vi "Vector space kNN.vi"() -> ()   [LabVIEW 2014]
uses:
  <vilib>/Utility/file.llb/Write To Spreadsheet File (string).vi
panel:
  out "Array 4":string[][](array[string])
  out "Slide 2":dbl(slide) scale=0.0..204.0
  out "Slide":dbl(slide) scale=0.0..9.0
  in  "Path":path
  in  "all rows":string[][](array[string])=array2038x3[6114 elements]
  out "LCS/min (Lsample,Lknown)":dbl[][](array[numeric])
  out "Distance values (LCS)":dbl[][](array[numeric])
  out "size(s)":i32
  out "accuracy":string[][](array[string])
  out "Results":string[][](array[string])
  out "Training data (K)":string[][](array[string])
  out "test data K-1":string[][](array[string])
  in  "K folds K":i32=10
  out "K folds data":string[][](array[string])
  out "Assigned using LCS (enhanced)":string[][](array[string])
  out "Assigned using LCS":string[][](array[string])
  in  "class labels for training data":string[](array[string])
  in  "kNN k":i32=5
  in  "training data (cluster centers)":string[](array[string])
  in  "test data (patterns in)":string[](array[string])=["0 4 0", "4 0 4", "0 4 0", "4 0 4", "0 4 0", "4 0 4", "0 4 0", "4 0 -2", "0 -2 3", "-2 3 0", "3 0 3", "0 3 0", "3 0 4", "0 4 0", "-2 0 1", "0 1 0", "1 0 -4", "0 -4 4", "-2 2 0", "2 0 -1", "0 -1 -4", "-1 -4 1", "-4 1 0", "1 0 3", "0 3 0", "-1 0 -1", "0 -1 2", "0 -1 1", "-1 1 0", "1 0 4", "0 4 0", "4 0 3", "0 3 -2", "3 -2 0", "-2 0 -2", "0 -2 3", "-2 3 -2", "3 -2 0", "-2 0 4", "0 4 0", "4 0 -2", "0 -2 2", "2 -1 0", "-1 0 4", "0 4 0", "4 0 2", "0 2 0", "2 0 -2", "0 -2 0", "1 -1 0", "-1 0 3", "0 3 0", "3 0 -4", "0 -4 4", "-4 4 -4", "4 -4 0", "2 -1 0", "-1 0 3", "0 3 -2", "3 -2 0", "-2 0 -3", "0 -3 0", "-3 0 3", "0 3 0", "3 0 -3", "0 -3 0", "0 4 0", "4 0 4", "0 4 -4", "4 -4 1", "-4 1 -1", "1 -1 0", "-1 0 -3", "0 -3 0", "-3 0 1", "0 1 -4", "1 -4 1", "-4 1 0", "1 0 4", "0 4 0", "4 0 -4", "0 -4 0", "-4 0 -4", "0 -4 4", "-4 4 -4", "4 -4 1", "0 -4 1", "-4 1 0", "1 0 -4", "0 -4 4", "0 4 0", "4 0 -2", "0 -2 2", "-2 2 -2", "2 -2 2", "-2 2 -2", "2 -2 2", "-2 2 -1", "2 -1 0", "-1 0 4", "0 4 0", "4 0 2", "0 2 0", "2 0 4", "0 4 0", "4 0 2", "0 2 -2", "2 -2 0", "-2 0 4", "1 0 -1", "0 -1 0", "-1 0 -1", "0 -1 0", "-1 0 1", "0 1 -1", "-2 2 -2", "2 -2 3", "1 0 -1", "0 -1 0", "-1 0 -1", "0 -1 2", "-1 2 0", "2 0 2", "0 2 -2", "2 -2 0", "-2 0 -4", "0 -4 0", "-2 2 0", "2 0 3", "0 3 -2", "3 -2 2", "1 -1 0", "-1 0 3", "0 4 0", "-2 0 1", "0 1 -4", "1 -4 0", "-4 0 -3", "0 -3 0", "1 0 -1", "0 -1 2", "-1 2 -1", "2 -1 1", "-1 1 -4", "-2 0 -1", "0 -1 1", "0 3 0", "3 0 3", "0 3 0", "3 0 3", "0 3 -2", "-4 0 -4", "0 -4 4", "0 4 0", "4 0 -4", "0 -4 0", "-4 0 -4", "-2 2 0", "2 0 4", "0 4 -4", "4 -4 0", "-4 0 2", "0 2 -2"]
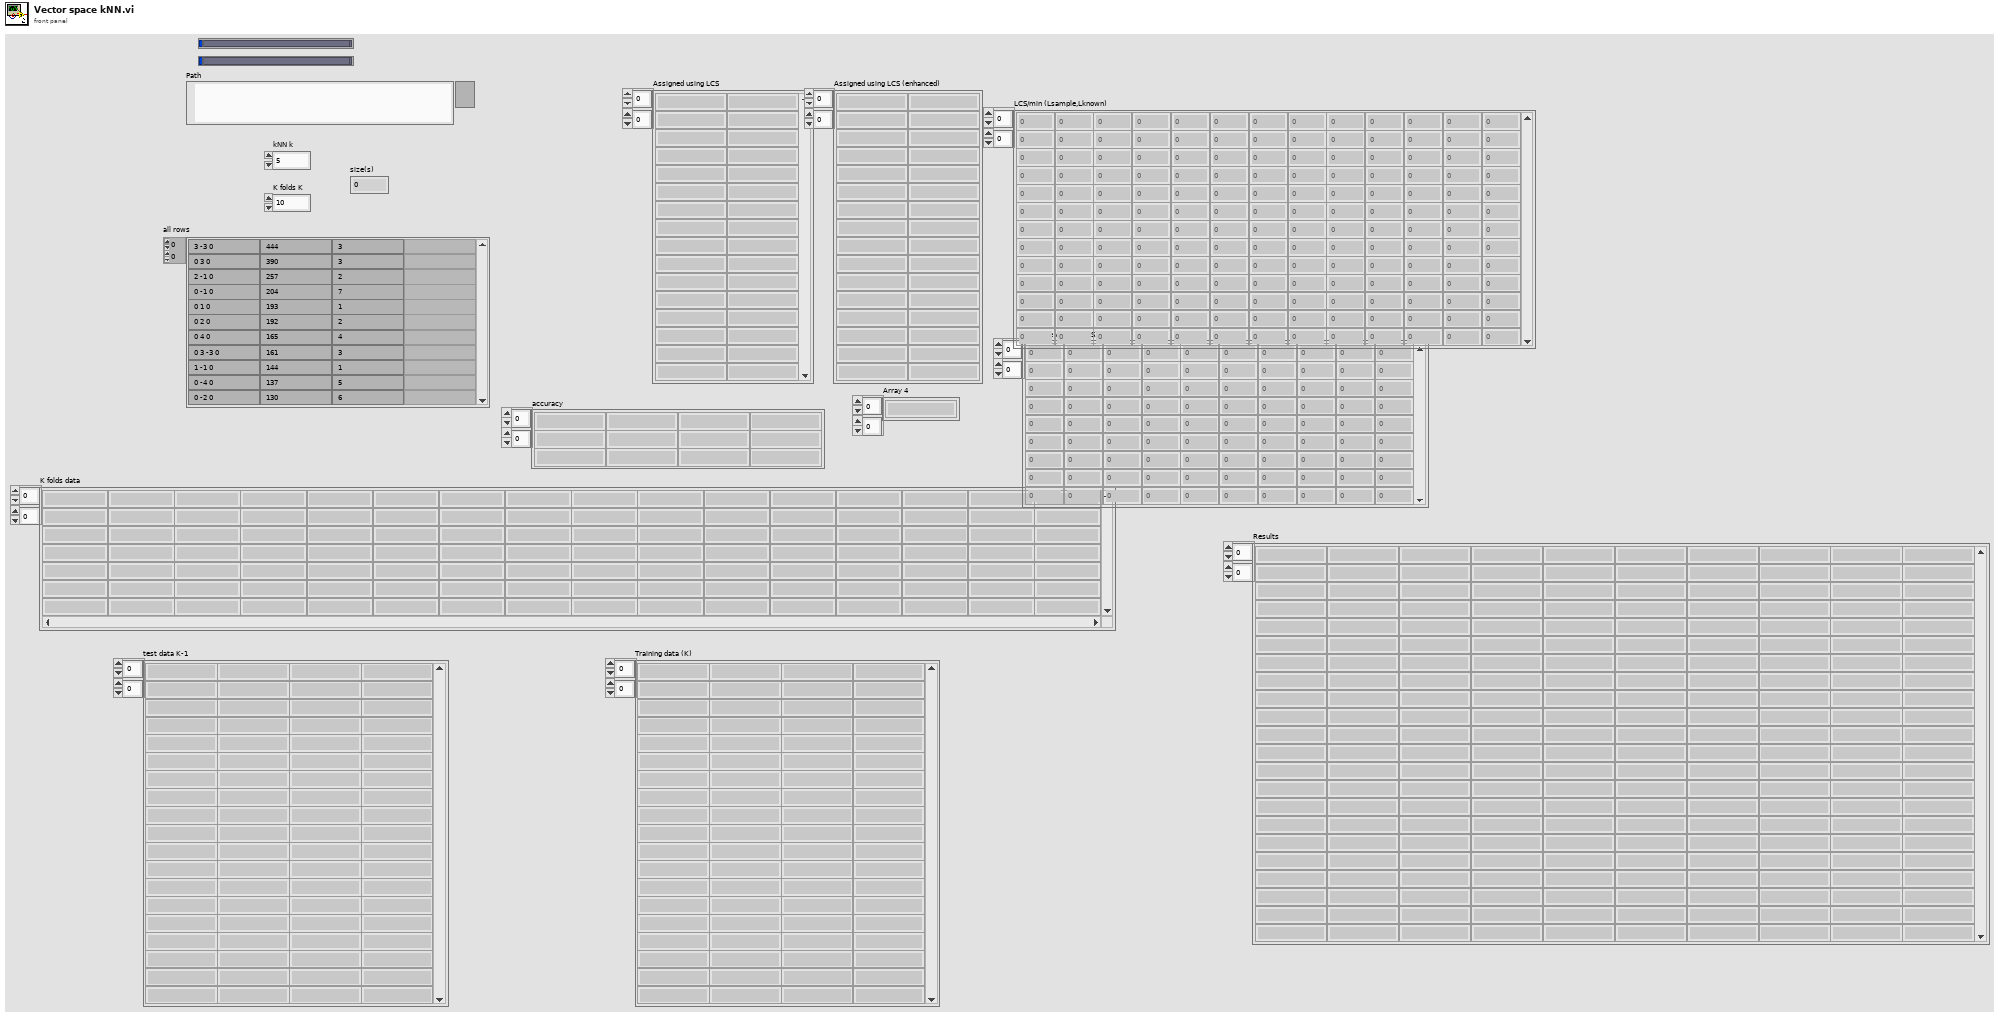
[diagram p1: front panel]
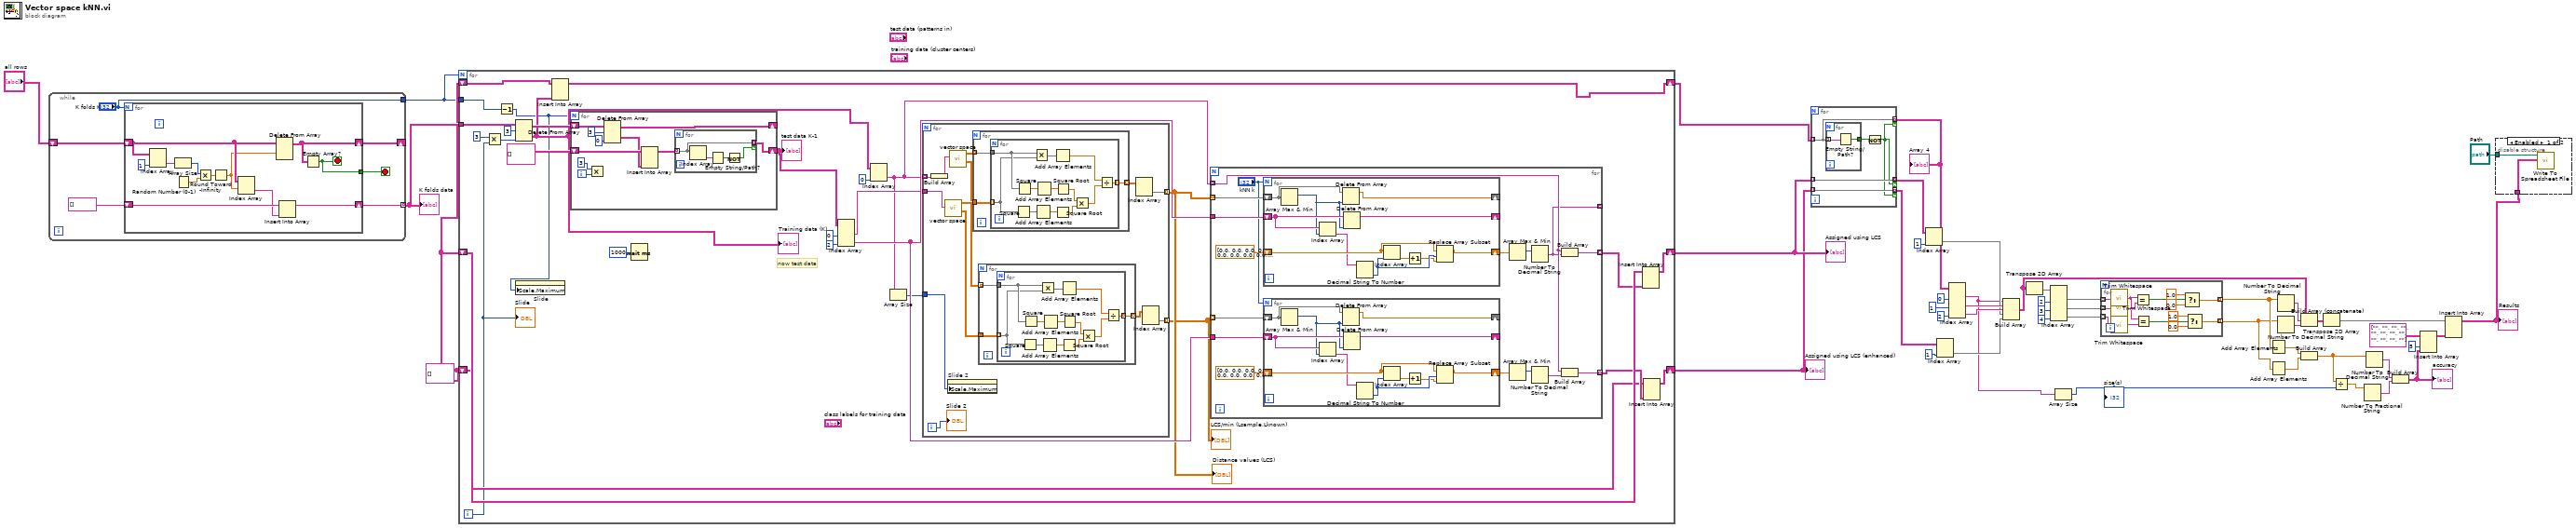
[diagram p0: block diagram]
diagram:
  w10 = string[][] []
  n1 = while {
    shift-right: [w50] -> _
    shift-left: "all rows" -> [w51]
    tunnel: [w52] -> w47 mode=indexing
    tunnel: ["K folds K"] -> w9
    stop <- w49 stop-if-true
    n2 = for {
      N: "K folds K" -> [_]
      shift-right: [w58] -> w52
      shift-left: string[] [] ("all rows 2") -> [w65]
      shift-right: [w56] -> w50
      shift-left: w51 -> [w57]
      tunnel: [w55] -> w49
      stop <- w55 stop-if-true
      n3 = Index Array(array=w57, index (col)=1 ("disabled index (col)")) -> (element=w61:string[])  [unwired: 1 in]
      n4 = Array Size(array=w61) -> (size(s)=w62:i32)
      n5 = Random Number (0-1)() -> (number: 0 to 1=w63:dbl)
      n6 = Multiply(x=w62, y=w63) -> (x*y=w64:dbl)
      n7 = Round Toward -Infinity(1:w64) -> (0:w54:dbl)
      n8 = Index Array(array=w57, index (row)=w54) -> (element=w59:string[])  [unwired: 1 in]
      n9 = Delete From Array(array=w57, index (row)=w54) -> (array with subset deleted=w56:string[][])  [unwired: 2 in, 1 out]
      n10 = Insert Into Array(array=w65, new element=w59) -> (w58:string[])  [unwired: 1 in]
      n11 = Empty Array?(array=w56) -> (empty?=w55:bool)
    }
  }
  "K folds data" <- w47
  n12 = for {
    N: w9 -> [_]
    tunnel: w47 -> [w94]
    tunnel: w9 -> [w70]
    shift-right: [w77] -> w6
    shift-left: w10 -> [w79]
    shift-right: [w74] -> w5
    shift-left: w10 -> [w76]
    shift-right: [w71] -> w3
    shift-left: w10 -> [w72]
    i -> [w69]
    # "now test data"
    n13 = Multiply(x=3, y=w69) -> (x*y=w83:i32)
    n14 = Decrement(x=w70) -> (x-1=w66:i32)
    n15 = Delete From Array(array=w94, length=3, index (col)=w83) -> (deleted portion=w78:string[][], array with subset deleted=w82:string[][])  [unwired: 1 in]
    "Training data (K)" <- w78
    n16 = property on="Slide" class="Slide (strict)"("Scale.Maximum"=w66) -> ()  [unwired: 2 in, 2 out]
    n17 = Insert Into Array(array=w79, new element=w78) -> (w77:string[][])  [unwired: 2 in]
    n18 = for {
      N: w66 -> [_]
      shift-right: [w95] -> w86
      shift-left: string[][] [] ("all rows 2") -> [w103]
      shift-right: [w98] -> _
      shift-left: w82 -> [w104]
      i -> [w100]
      n19 = Multiply(x=3, y=w100) -> ()  [unwired: 1 out]
      n20 = Delete From Array(array=w104, length=3 ("index (col)"), index (col)=0 ("disabled index (col)")) -> (deleted portion=w102:string[][], array with subset deleted=w98:string[][])  [unwired: 1 in]
      n21 = Insert Into Array(array=w103, new element=w102) -> (w96:string[][])  [unwired: 2 in]
      n22 = for {
        tunnel: w96 -> [w107] mode=indexing
        tunnel: [w107] -> w95 mode=indexing if=w108
        n23 = Index Array(array=w107) -> (element=w106:string)  [unwired: 1 in]
        n24 = Empty String/Path?(string/path=w106) -> (empty?=w105:bool)
        n25 = Not(x=w105) -> (.not. x?=w108:bool)
      }
    }
    "test data K-1" <- w86
    n26 = Wait (ms)(milliseconds to wait=u32 1000) -> ()  [unwired: 1 out]
    n27 = Index Array(array=w86, index (col) #1=0 ("disabled index (col)"), index (col) #2=2 ("index (col)")) -> (element #1=w89:string[], element #2=w90:string[])  [unwired: 2 in]
    n28 = Index Array(array=w78, index (col)=0 ("disabled index (col)")) -> (element=w68:string[])  [unwired: 1 in]
    n29 = Array Size(array=w68) -> (size(s)=w67:i32)
    n30 = for {
      tunnel: w68 -> [w159] mode=indexing
      tunnel: w89 -> [w154]
      tunnel: [w158] -> w88 mode=indexing
      tunnel: [w149] -> w87 mode=indexing
      tunnel: w67 -> [w147]
      i -> [w148]
      n31 = Build Array(w159) -> (w155:string[])
      n32 = call "vector space.vi"("Full transition sequence from service to end"=w154) -> ("vector (directional transitions)"=w151:dbl[][], "vector positions only"=w156:dbl[][])  [unwired: 8 in, 1 out]
      n33 = property on="Slide 2" class="Slide (strict)"("Scale.Maximum"=w147) -> ()  [unwired: 2 in, 2 out]
      n34 = call "vector space.vi"("Full transition sequence from service to end"=w155) -> ("vector (directional transitions)"=w152:dbl[][], "vector positions only"=w157:dbl[][])  [unwired: 8 in, 1 out]
      n35 = for {
        tunnel: w157 -> [w176] mode=indexing
        tunnel: w156 -> [w177]
        tunnel: [w175] -> w153 mode=indexing
        n36 = for {
          tunnel: w177 -> [w183] mode=indexing
          tunnel: w176 -> [w189]
          tunnel: [w178] -> w175 mode=indexing
          n37 = Square(x=w183) -> (x^2=w184:dbl[])
          n38 = Square(x=w189) -> (x^2=w187:dbl[])
          n39 = Multiply(x=w189, y=w183) -> (x*y=w188:dbl[])
          n40 = Add Array Elements(numeric array=w184) -> (sum=w185:dbl)
          n41 = Add Array Elements(numeric array=w187) -> (sum=w186:dbl)
          n42 = Add Array Elements(numeric array=w188) -> (sum=w179:dbl)
          n43 = Square Root(x=w185) -> (sqrt(x)=w181:dbl)
          n44 = Square Root(x=w186) -> (sqrt(x)=w182:dbl)
          n45 = Multiply(x=w182, y=w181) -> (x*y=w180:dbl)
          n46 = Divide(x=w179, y=w180) -> (x/y=w178:dbl)
        }
      }
      n47 = for {
        tunnel: w152 -> [w161] mode=indexing
        tunnel: w151 -> [w162]
        tunnel: [w160] -> w150 mode=indexing
        n48 = for {
          tunnel: w162 -> [w168] mode=indexing
          tunnel: w161 -> [w174]
          tunnel: [w163] -> w160 mode=indexing
          n49 = Square(x=w168) -> (x^2=w169:dbl[])
          n50 = Square(x=w174) -> (x^2=w172:dbl[])
          n51 = Multiply(x=w174, y=w168) -> (x*y=w173:dbl[])
          n52 = Add Array Elements(numeric array=w169) -> (sum=w170:dbl)
          n53 = Add Array Elements(numeric array=w172) -> (sum=w171:dbl)
          n54 = Add Array Elements(numeric array=w173) -> (sum=w164:dbl)
          n55 = Square Root(x=w170) -> (sqrt(x)=w166:dbl)
          n56 = Square Root(x=w171) -> (sqrt(x)=w167:dbl)
          n57 = Multiply(x=w167, y=w166) -> (x*y=w165:dbl)
          n58 = Divide(x=w164, y=w165) -> (x/y=w163:dbl)
        }
      }
      n59 = Index Array(array=w153) -> (element=w158:dbl[])  [unwired: 2 in]
      n60 = Index Array(array=w150) -> (element=w149:dbl[])  [unwired: 2 in]
      "Slide 2" <- w148
    }
    "Distance values (LCS)" <- w88
    "LCS/min (Lsample,Lknown)" <- w87
    n61 = for {
      tunnel: w68 -> [w115] mode=indexing
      tunnel: w88 -> [w124] mode=indexing
      tunnel: w90 -> [w123]
      tunnel: w87 -> [w114] mode=indexing
      tunnel: w90 -> [w113]
      tunnel: [w112] -> w75 mode=indexing
      tunnel: [w111] -> w73 mode=indexing
      tunnel: [w109] -> _ mode=indexing
      n62 = for {
        N: "kNN k" -> [_]
        shift-right: [w143] -> _
        shift-left: w124 -> [w146]
        shift-right: [w142] -> _
        shift-left: w123 -> [w145]
        shift-right: [w137] -> w120
        shift-left: dbl[] [0.0, 0.0, 0.0, 0.0, 0.0, 0.0, 0.0, 0.0, 0.0, 0.0, 0.0, 0.0] -> [w138]
        n63 = Array Max & Min(array=w146) -> (max index (indices)=w144:i32)  [unwired: 3 out]
        n64 = Index Array(array=w145, index=w144) -> (element=w136:string)
        n65 = Delete From Array(array=w146, index=w144) -> (array with subset deleted=w143:dbl[])  [unwired: 1 in, 1 out]
        n66 = Delete From Array(array=w145, index=w144) -> (array with subset deleted=w142:string[])  [unwired: 1 in, 1 out]
        n67 = Decimal String To Number(string=w136) -> (number=w141:i32)  [unwired: 2 in, 1 out]
        n68 = Index Array(array=w138, index=w141) -> (element=w139:dbl)
        n69 = Increment(x=w139) -> (x+1=w140:dbl)
        n70 = Replace Array Subset(array=w138, new element=w140, index=w141) -> (w137:dbl[])
      }
      n71 = for {
        N: "kNN k" -> [_]
        shift-right: [w132] -> _
        shift-left: w114 -> [w135]
        shift-right: [w131] -> _
        shift-left: w113 -> [w134]
        shift-right: [w126] -> w118
        shift-left: dbl[] [0.0, 0.0, 0.0, 0.0, 0.0, 0.0, 0.0, 0.0, 0.0, 0.0, 0.0, 0.0] -> [w127]
        n72 = Array Max & Min(array=w135) -> (max index (indices)=w133:i32)  [unwired: 3 out]
        n73 = Index Array(array=w134, index=w133) -> (element=w125:string)
        n74 = Delete From Array(array=w135, index=w133) -> (array with subset deleted=w132:dbl[])  [unwired: 1 in, 1 out]
        n75 = Delete From Array(array=w134, index=w133) -> (array with subset deleted=w131:string[])  [unwired: 1 in, 1 out]
        n76 = Decimal String To Number(string=w125) -> (number=w130:i32)  [unwired: 2 in, 1 out]
        n77 = Index Array(array=w127, index=w130) -> (element=w128:dbl)
        n78 = Increment(x=w128) -> (x+1=w129:dbl)
        n79 = Replace Array Subset(array=w127, new element=w129, index=w130) -> (w126:dbl[])
      }
      n80 = Array Max & Min(array=w120) -> (max index (indices)=w121:i32)  [unwired: 3 out]
      n81 = Array Max & Min(array=w118) -> (max index (indices)=w117:i32)  [unwired: 3 out]
      n82 = Number To Decimal String(number=w121) -> (decimal integer string=w109:string)  [unwired: 1 in]
      n83 = Number To Decimal String(number=w117) -> (decimal integer string=w119:string)  [unwired: 1 in]
      n84 = Build Array(w115, w109) -> (w112:string[])
      n85 = Build Array(w115, w119) -> (w111:string[])
    }
    n86 = Insert Into Array(array=w76, new element=w75) -> (w74:string[][])  [unwired: 2 in]
    n87 = Insert Into Array(array=w72, new element=w73) -> (w71:string[][])  [unwired: 2 in]
    "Slide" <- w69
  }
  "Assigned using LCS" <- w5
  "Assigned using LCS (enhanced)" <- w3
  n88 = for {
    tunnel: w6 -> [w193] mode=indexing
    tunnel: [w193] -> w4 mode=indexing if=w190
    tunnel: w5 -> [w192] mode=indexing
    tunnel: [w192] -> w1 mode=indexing if=w190
    tunnel: [w191] -> w2 mode=indexing if=w190
    tunnel: w3 -> [w191] mode=indexing
    n89 = for {
      tunnel: w193 -> [w196] mode=indexing
      tunnel: [w195] -> w194
      n90 = Empty String/Path?(string/path=w196) -> (empty?=w195:bool)
    }
    n91 = Not(x=w194) -> (.not. x?=w190:bool)
  }
  "Array 4" <- w4
  n92 = Index Array(array=w1, index (col)=1 ("disabled index (col)")) -> (element=w17:string[])  [unwired: 1 in]
  n93 = Index Array(array=w2, index (col)=1 ("disabled index (col)")) -> (element=w15:string[])  [unwired: 1 in]
  n94 = Index Array(array=w4, index (col) #1=0 ("disabled index (col)"), index (col) #2=1 ("index (col)"), index (col) #3=2 ("index (col)")) -> (element #1=w13:string[], element #2=w20:string[], element #3=w19:string[])  [unwired: 3 in]
  n95 = Build Array(w13, w20, w19, w17, w15) -> (w14:string[][])
  n96 = Transpose 2D Array(2D array=w14) -> (transposed array=w38:string[][])
  n97 = Index Array(array=w38, index (col) #1=2 ("disabled index (col)"), index (col) #2=3 ("index (col)"), index (col) #3=4 ("index (col)")) -> (element #1=w41:string[], element #2=w40:string[], element #3=w39:string[])  [unwired: 3 in]
  n98 = Array Size(array=w13) -> (size(s)=w12:i32)
  "size(s)" <- w12
  n99 = for {
    tunnel: w41 -> [w202] mode=indexing
    tunnel: w40 -> [w201] mode=indexing
    tunnel: w39 -> [w200] mode=indexing
    tunnel: [w204] -> w23 mode=indexing
    tunnel: [w203] -> w22 mode=indexing
    n100 = call <vilib>:"Trim Whitespace.vi"("string"=w201) -> ("trimmed string"=w199:string)  [unwired: 1 in]
    n101 = call <vilib>:"Trim Whitespace.vi"("string"=w200) -> ("trimmed string"=w198:string)  [unwired: 1 in]
    n102 = call <vilib>:"Trim Whitespace.vi"("string"=w202) -> ("trimmed string"=w197:string)  [unwired: 1 in]
    n103 = Equal?(x=w197, y=w199) -> (x = y?=w210:bool)
    n104 = Equal?(x=w197, y=w198) -> (x = y?=w205:bool)
    n105 = Select(t=1.0, s=w210, f=0.0) -> (s? t:f=w204:dbl)
    n106 = Select(t=1.0, s=w205, f=0.0) -> (s? t:f=w203:dbl)
  }
  n107 = Add Array Elements(numeric array=w23) -> (sum=w24:dbl)
  n108 = Add Array Elements(numeric array=w22) -> (sum=w25:dbl)
  n109 = Number To Decimal String(number=w23) -> (decimal integer string=w37:string[])  [unwired: 1 in]
  n110 = Number To Decimal String(number=w22) -> (decimal integer string=w36:string[])  [unwired: 1 in]
  n111 = Build Array (concatenate)(w14, w37, w36) -> (w35:string[][])
  n112 = Build Array(w24, w25) -> (w26:dbl[])
  n113 = Transpose 2D Array(2D array=w35) -> (transposed array=w21:string[][])
  n114 = Divide(x=w26, y=w12) -> (x/y=w27:dbl[])
  n115 = Number To Fractional String(number=w27) -> (F-format string=w29:string[])  [unwired: 3 in]
  n116 = Number To Decimal String(number=w26) -> (decimal integer string=w28:string[])  [unwired: 1 in]
  n117 = Build Array(w28, w29) -> (w33:string[][])
  "accuracy" <- w33
  n118 = Insert Into Array(array=string[][] [["", "", "", "", "", ""], ["", "", "", "", "", ""]] ("appended array 3"), index (col)=5 ("disabled index (col)"), new element=w33) -> (w32:string[][])  [unwired: 1 in]
  n119 = Insert Into Array(array=w21, new element=w32) -> (w8:string[][])  [unwired: 2 in]
  "Results" <- w8
  n120 = disable-structure shown="Enabled" {
    disable-tunnel: "Path" -> [w212 _]
    disable-tunnel: w8 -> [w211 _]
    frame Enabled {
      n121 = call-poly <vilib>:"Write To Spreadsheet File.vi"("2D data"=w211, "file path (dialog if empty)"=w212) -> ()  [unwired: 6 in, 1 out]
    }
    frame Disabled {
    }
  }
